vi "SVA 4MV6 PF CCE MGLD PMJD.vi"() -> ()   [LabVIEW 2020]
uses:
  <vilib>/userDefined/High Color/IMAQdx.ctl
  SVA 4MV6 PF CCE MGLD PMJD.ctl
  <vilib>/vision/driver/IMAQdx.llb/IMAQdx Buffer Number Mode.ctl
  <vilib>/vision/driver/NI_Vision_Acquisition_Software.lvlib
panel:
  out "Sin abolladuras":bool
  out "Etiqueta detectada":bool
  out "Orientacion etiqueta correcta":bool
  out "Pass Status":bool
  out "Tapa y etiqueta correctas":bool
  out "Color 2":u32(colorbox)
  out "Color":u32(colorbox)
  out "Color etiqueta":string
  out "Color tapa":string
  out "Nivel de liquido":bool[](array[boolean])
  out "Tapa detectada":bool
  out "Entrada de video":T1(plugin-control)
  out "captura":T1(plugin-control)
  in  "capturar imagen":bool
  in  "stop":bool
  in  "Session In":T2="cam1"
  # "Ceballos Conde Emanuel  Meneses Gutiérrez Luis David  Pineda Méndez Job Daniel\n                            4MV6 Sistemas de vision artificial  Proyecto Final"
  # "Condiciones para Aceptar el producto:\n-Detectar tapa y etiqueta \n-Color de tapa y etiqueta iguales\n-Orientacion de la etiqueta correcta\n-Nivel de liquido dentro del rango maximo\n-Botella sin abolladuras"
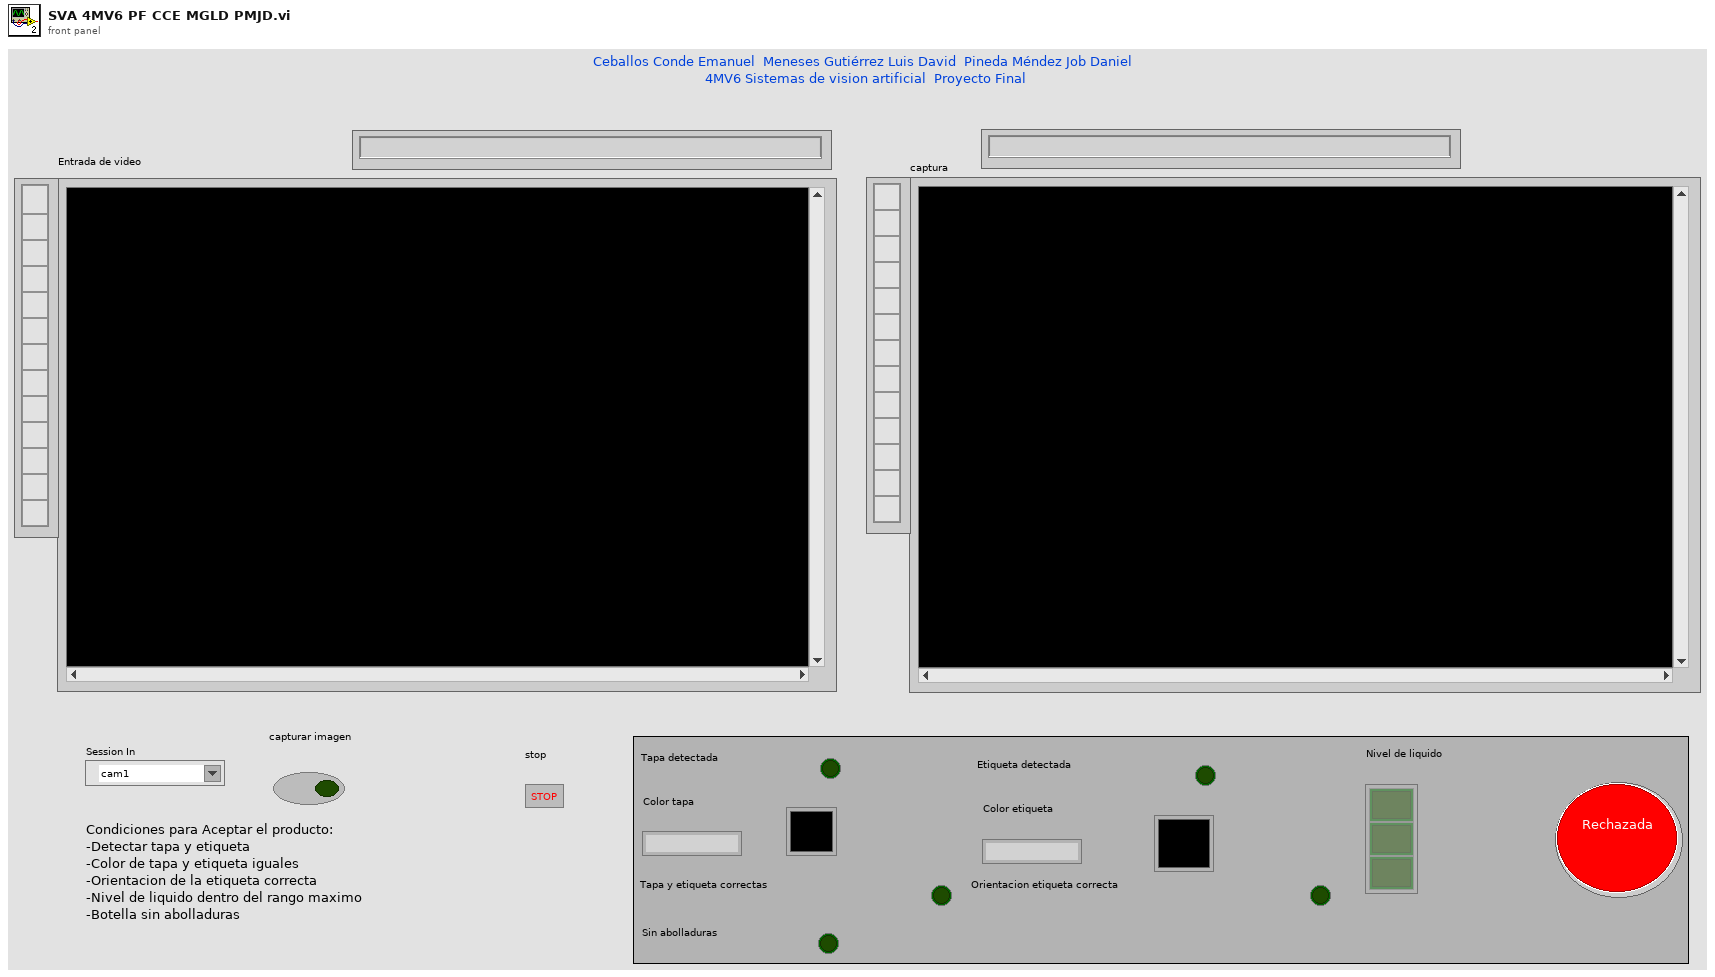
[diagram p1: front panel]
types:
  T1 = typedef "IMAQ Image.ctl" = refnum<image>
  T2 = typedef "IMAQdx.ctl" = refnum<k21>
  T3 = typedef "Image Type" = u32
  T4 = typedef "SVA 4MV6 PF CCE MGLD PMJD.ctl" = enum16{"espera", "captura", "tapa ", "etiqueta", "color", "nivel", "forma", "aceptar"}
  T5 = typedef "NI_Vision_Acquisition_Software.lvlib/IMAQdx Buffer Number Mode.ctl" = enum32{"Next", "Last", "Buffer Number", "Every", "Last New"}
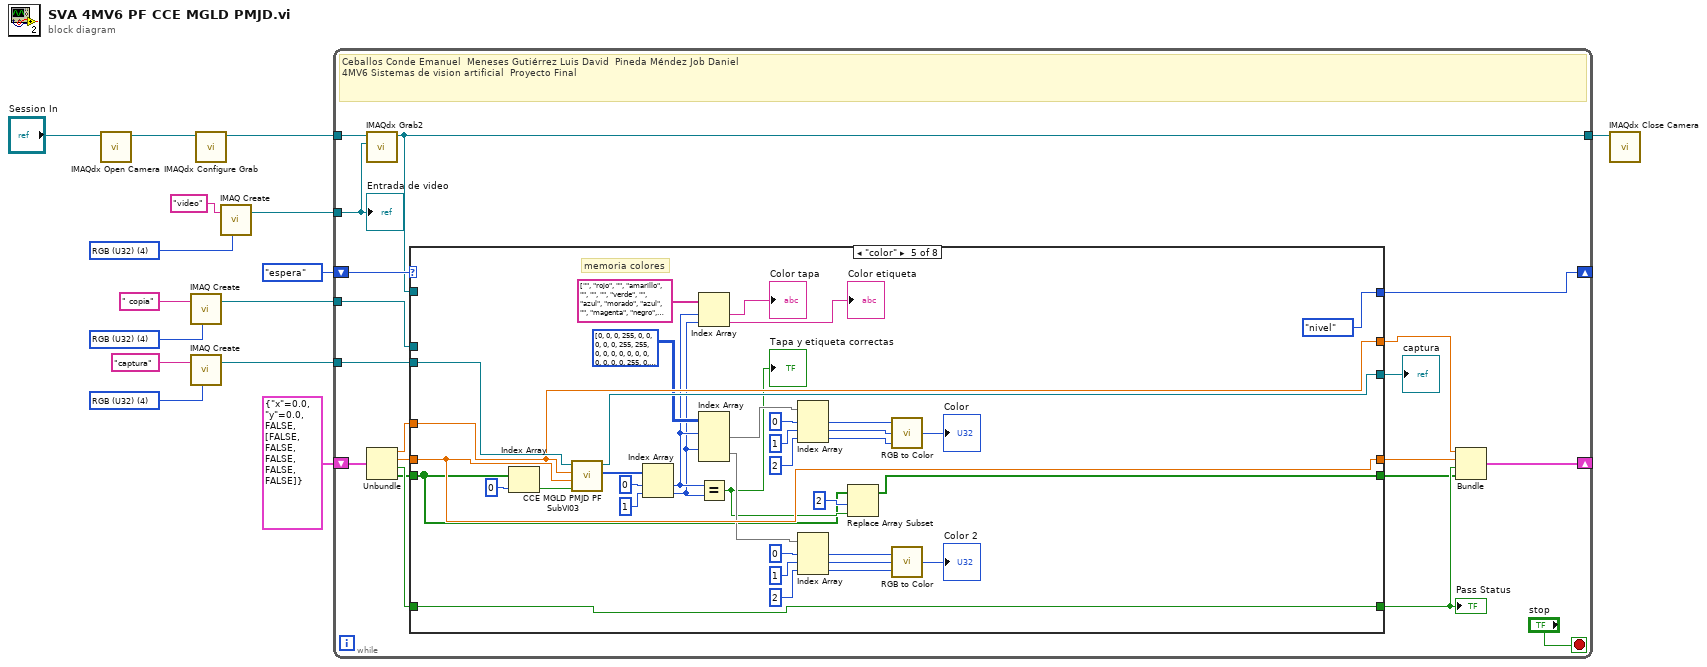
[diagram p0: block diagram]
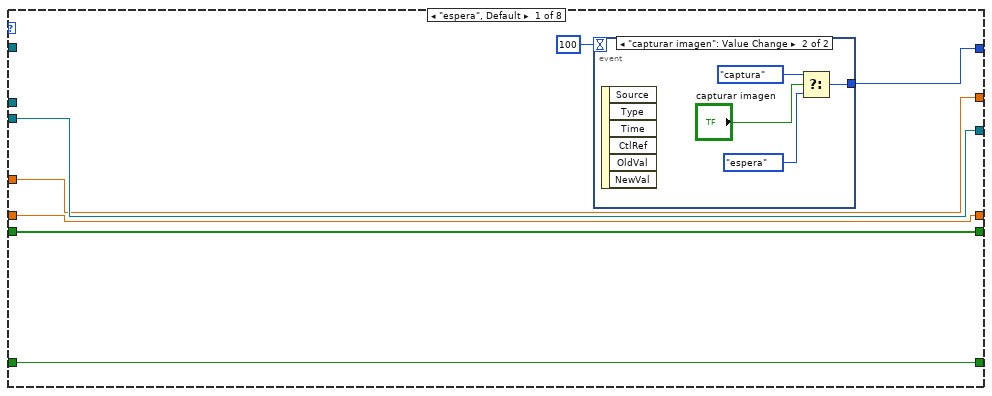
[diagram p2: hidden frame]
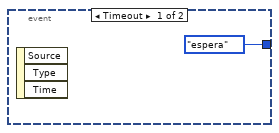
[diagram p3: hidden frame]
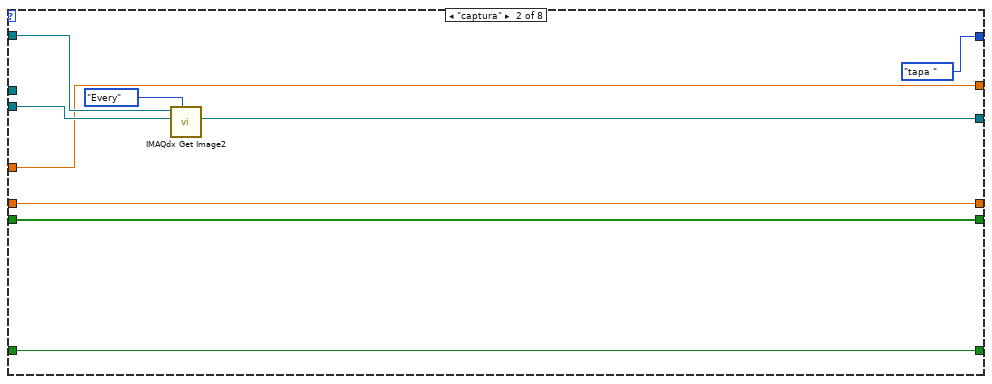
[diagram p4: hidden frame]
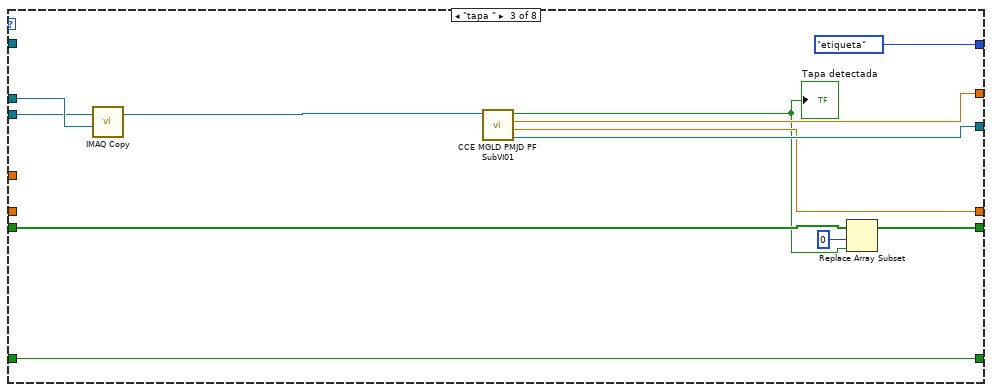
[diagram p5: hidden frame]
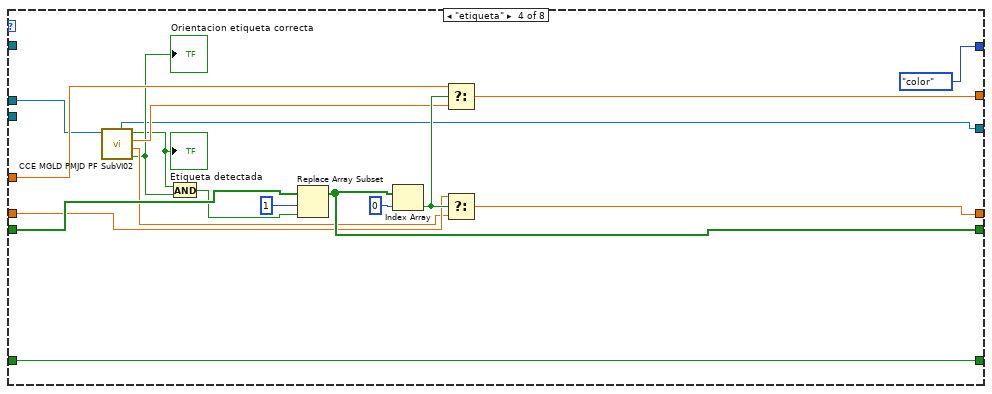
[diagram p6: hidden frame]
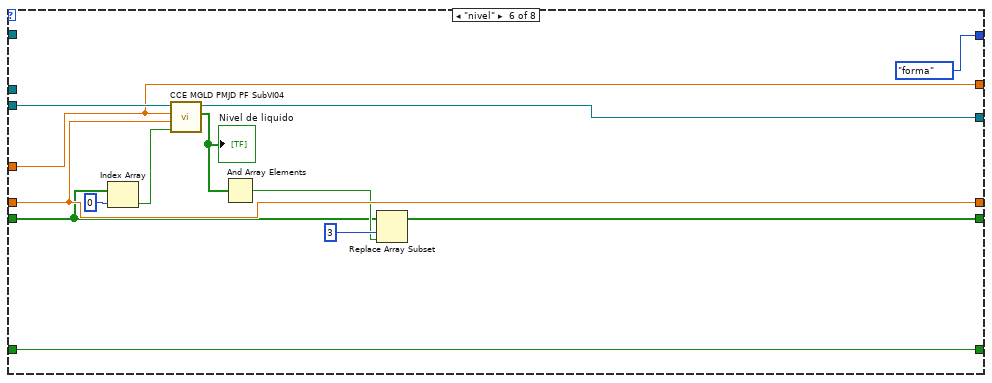
[diagram p7: hidden frame]
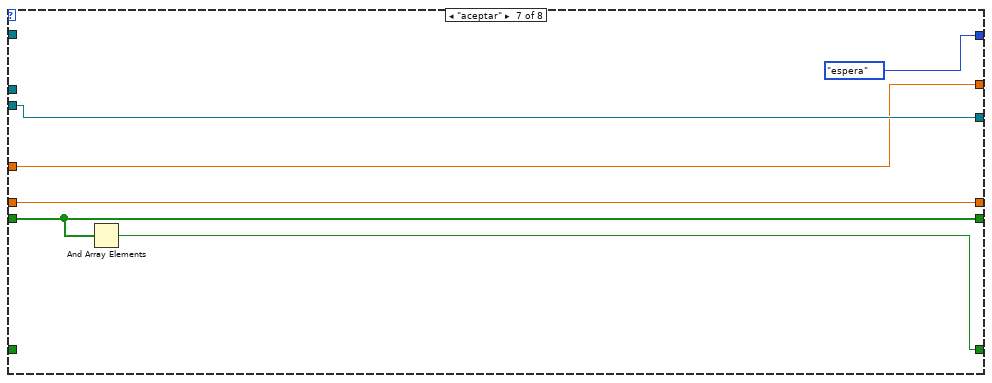
[diagram p8: hidden frame]
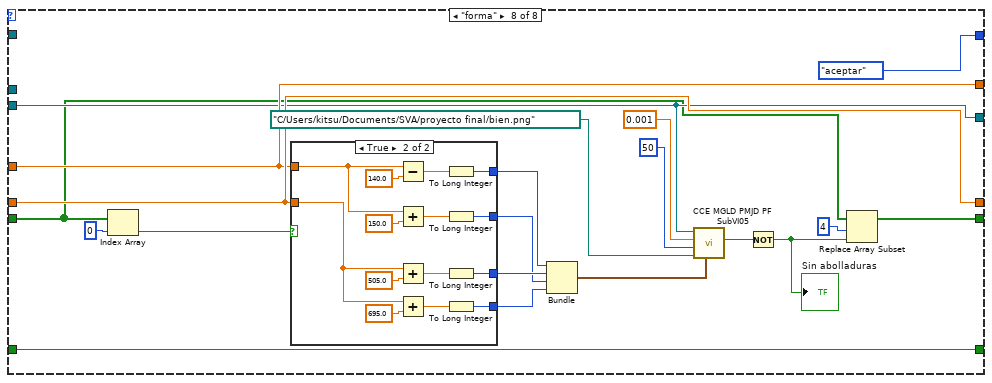
[diagram p9: hidden frame]
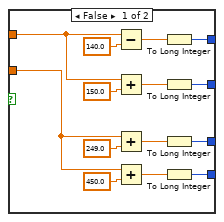
[diagram p10: hidden frame]
diagram:
  w3 = T3 4 items=["Grayscale (U8)", "Grayscale (I16)", "Grayscale (SGL)", "Complex (CSG)", "RGB (U32)", "HSL (U32)", "RGB (U64)", "Grayscale (U16)"] ("Image Type")
  w10 = T3 4 items=["Grayscale (U8)", "Grayscale (I16)", "Grayscale (SGL)", "Complex (CSG)", "RGB (U32)", "HSL (U32)", "RGB (U64)", "Grayscale (U16)"] ("Image Type")
  w12 = T3 4 items=["Grayscale (U8)", "Grayscale (I16)", "Grayscale (SGL)", "Complex (CSG)", "RGB (U32)", "HSL (U32)", "RGB (U64)", "Grayscale (U16)"] ("Image Type")
  n1 = call <vilib>:"IMAQdx Open Camera.vi"("Session In"="Session In") -> ("Session Out"=w14:T2)  [unwired: 9 in, 1 out]
  n2 = call "IMAQ Create"("Image Name"=" copia", "Image Type"=w3) -> ("New Image"=w2:T1)  [unwired: 3 in, 1 out]
  n3 = call "IMAQ Create"("Image Name"="captura", "Image Type"=w12) -> ("New Image"=w5:T1)  [unwired: 3 in, 1 out]
  n4 = call <vilib>:"IMAQdx Configure Grab.vi"("Session In"=w14) -> ("Session Out"=w7:T2)  [unwired: 9 in, 1 out]
  n5 = call "IMAQ Create"("Image Name"="video", "Image Type"=w10) -> ("New Image"=w8:T1)  [unwired: 3 in, 1 out]
  n6 = while {
    shift-right: [w33] -> _
    shift-left: SVA_4MV6_PF_CCE_MGLD_PMJD."espera" -> [w34]
    tunnel: w8 -> [w28]
    tunnel: w7 -> [w32]
    tunnel: [w31] -> w6
    tunnel: w5 -> [w29]
    tunnel: w2 -> [w27]
    shift-right: [w26] -> _
    shift-left: cluster{"x":sgl, "y":sgl, bool, bool[]} {"x"=0.0, "y"=0.0, FALSE, [FALSE, FALSE, FALSE, FALSE, FALSE]} -> [w25]
    stop <- "stop" stop-if-true
    # "Ceballos Conde Emanuel  Meneses Gutiérrez Luis David  Pineda Méndez Job Daniel\n4MV6 Sistemas de vision artificial  Proyecto Final"
    n7 = call <vilib>:"IMAQdx Grab2.vi"("Image In"=w28, "Session In"=w32) -> ("Session Out"=w31:T2)  [unwired: 6 in, 3 out]
    n8 = Unbundle(w25) -> ("x"=w24:sgl, "y"=w23:sgl, w19:bool, w18:bool[])
    n9 = case shown="\"color\"" w34 {
      tunnel: [w40 SVA_4MV6_PF_CCE_MGLD_PMJD."tapa " SVA_4MV6_PF_CCE_MGLD_PMJD."etiqueta" SVA_4MV6_PF_CCE_MGLD_PMJD."color" SVA_4MV6_PF_CCE_MGLD_PMJD."nivel" SVA_4MV6_PF_CCE_MGLD_PMJD."forma" SVA_4MV6_PF_CCE_MGLD_PMJD."espera" SVA_4MV6_PF_CCE_MGLD_PMJD."aceptar"] -> w33
      tunnel: w31 -> [_ w54 _ _ _ _ _ _]
      tunnel: [w39 w53 w66 w70 w121 w132 w140 w150] -> w30
      tunnel: w29 -> [w39 w52 w64 _ w122 w135 w140 w150]
      tunnel: w27 -> [_ _ w65 w71 _ _ _ _]
      tunnel: [w38 w50 w63 w69 w120 w134 w139 w151] -> w22
      tunnel: [w37 w49 w62 w83 w119 w133 w138 w152] -> w21
      tunnel: w24 -> [w38 w50 _ w79 w120 w134 w139 w151]
      tunnel: w23 -> [w37 w49 _ w78 w119 w133 w138 w152]
      tunnel: [w36 w48 w61 w68 w93 w130 w137 w153] -> w20
      tunnel: w19 -> [w36 w48 w61 w68 w93 w130 _ w153]
      tunnel: w18 -> [w35 w47 w60 w84 w88 w124 w136 w143]
      tunnel: [w35 w47 w57 w81 w91 w127 w136 w147] -> w17
      frame "espera", Default {
        n10 = event shown="[1] \"capturar imagen\": Value Change" {
          selector: _ -> [_ _]
          dyn-events: _ -> [_ _]
          timeout: 100 -> [_ _]
          tunnel: [SVA_4MV6_PF_CCE_MGLD_PMJD."espera" w45] -> w40
          event Timeout {
            n11 = event-data() -> ()  [unwired: 1 in, 3 out]
          }
          event "capturar imagen": Value Change {
            n12 = event-data() -> ()  [unwired: 1 in, 6 out]
            n13 = Select(t=SVA_4MV6_PF_CCE_MGLD_PMJD."captura", s="capturar imagen", f=SVA_4MV6_PF_CCE_MGLD_PMJD."espera") -> (s? t:f=w45:T4)
          }
        }
      }
      frame "captura" {
        n14 = call <vilib>:"IMAQdx Get Image2.vi"("Buffer Number Mode (Next)"=IMAQdx_Buffer_Number_Mode."Every", "Image In"=w52, "Session In"=w54) -> ("Image Out"=w53:T1)  [unwired: 5 in, 3 out]
      }
      frame "tapa " {
        n15 = call "IMAQ Copy"("Image Dst"=w65, "Image Src"=w64) -> ("Image Dst Out"=w67:T1)  [unwired: 4 in, 1 out]
        n16 = call "CCE MGLD PMJD PF SubVI01.vi"("captura"=w67) -> ("Image 4"=w66:T1, "y"=w62:sgl, "x"=w63:sgl, "tapa detectada"=w59:bool)  [unwired: 7 in]
        "Tapa detectada" <- w59
        n17 = Replace Array Subset(array=w60, new element=w59, index=0) -> (w57:bool[])
      }
      frame "etiqueta" {
        n18 = call "CCE MGLD PMJD PF SubVI02.vi"("captura"=w71) -> ("orientacion correcta"=w75:bool, "y"=w76:sgl, "x"=w77:sgl, "etiqueta detectada"=w74:bool, "Image 4"=w70:T1)  [unwired: 6 in]
        "Orientacion etiqueta correcta" <- w75
        "Etiqueta detectada" <- w74
        n19 = And(x=w74, y=w75) -> (x .and. y?=w73:bool)
        n20 = Replace Array Subset(array=w84, new element=w73, index=1) -> (w81:bool[])
        n21 = Index Array(array=w81, index=0) -> (element=w82:bool)
        n22 = Select(t=w79, s=w82, f=w77) -> (s? t:f=w69:sgl)
        n23 = Select(t=w78, s=w82, f=w76) -> (s? t:f=w83:sgl)
      }
      frame "color" {
        # "memoria colores"
        n24 = Index Array(array=w88, index=0) -> (element=w87:bool)
        n25 = call "CCE MGLD PMJD PF SubVI03.vi"("tapa?"=w87, "y"=w119, "x"=w120, "Image 2"=w122) -> ("Array"=w94:i32[], "Image"=w121:T1)  [unwired: 6 in]
        n26 = Index Array(array=w94, index #1=0 ("index"), index #2=1 ("index")) -> (element #1=w96:i32, element #2=w95:i32)
        n27 = Index Array(array=string[] ["", "rojo", "", "amarillo", "", "", "", "verde", "", "azul", "morado", "azul", "", "magenta", "negro", "blanco"], index #1=w96, index #2=w95) -> (element #1=→"Color tapa":string, element #2=→"Color etiqueta":string)
        n28 = Index Array(array=u8[][] [[0, 0, 0], [255, 0, 0], [0, 0, 0], [255, 255, 0], [0, 0, 0], [0, 0, 0], [0, 0, 0], [0, 255, 0], [0, 0, 0], [0, 0, 255], [255, 0, 255], [0, 0, 255], [0, 0, 0], [255, 0, 255], [0, 0, 0], [255, 255, 255]], index (row) #1=w96, index (row) #2=w95) -> (element #1=w112:u8[], element #2=w111:u8[])  [unwired: 2 in]
        n29 = Equal?(x=w96, y=w95) -> (x = y?=w90:bool)
        "Tapa y etiqueta correctas" <- w90
        n30 = Index Array(array=w112, index #1=0 ("index"), index #2=1 ("index"), index #3=2 ("index")) -> (element #1=w103:u8, element #2=w102:u8, element #3=w101:u8)
        n31 = Index Array(array=w111, index #1=0 ("index"), index #2=1 ("index"), index #3=2 ("index")) -> (element #1=w99:u8, element #2=w98:u8, element #3=w97:u8)
        n32 = Replace Array Subset(array=w88, new element=w90, index=2) -> (w91:bool[])
        n33 = call <vilib>:"RGB to Color.vi"("B"=w101, "G"=w102, "R"=w103) -> ("Color"=→"Color":u32)
        n34 = call <vilib>:"RGB to Color.vi"("B"=w97, "G"=w98, "R"=w99) -> ("Color"=→"Color 2":u32)
      }
      frame "nivel" {
        n35 = Index Array(array=w124, index=0) -> (element=w125:bool)
        n36 = call "CCE MGLD PMJD PF SubVI04.vi"("tapa?"=w125, "y"=w133, "x"=w134, "Image 2"=w135) -> ("Array"=w131:bool[], "Image"=w132:T1)  [unwired: 6 in]
        "Nivel de liquido" <- w131
        n37 = And Array Elements(Boolean array=w131) -> (logical AND=w128:bool)
        n38 = Replace Array Subset(array=w124, new element=w128, index=3) -> (w127:bool[])
      }
      frame "aceptar" {
        n39 = And Array Elements(Boolean array=w136) -> (logical AND=w137:bool)
      }
      frame "forma" {
        n40 = Index Array(array=w143, index=0) -> (element=w142:bool)
        n41 = case shown="True" w142 {
          tunnel: [w171 w185] -> w161
          tunnel: [w166 w180] -> w160
          tunnel: [w165 w179] -> w159
          tunnel: [w164 w178] -> w158
          tunnel: w152 -> [w163 w177]
          tunnel: w151 -> [w162 w176]
          frame False {
            n42 = Subtract(x=w162, y=sgl 140.0) -> (x-y=w175:sgl)
            n43 = Add(x=w162, y=sgl 150.0) -> (x+y=w172:sgl)
            n44 = Add(x=w163, y=sgl 249.0) -> (x+y=w174:sgl)
            n45 = Add(x=w163, y=sgl 450.0) -> (x+y=w173:sgl)
            n46 = To Long Integer(number=w175) -> (32bit integer=w171:i32)
            n47 = To Long Integer(number=w172) -> (32bit integer=w165:i32)
            n48 = To Long Integer(number=w174) -> (32bit integer=w166:i32)
            n49 = To Long Integer(number=w173) -> (32bit integer=w164:i32)
          }
          frame True {
            n50 = Subtract(x=w176, y=sgl 140.0) -> (x-y=w189:sgl)
            n51 = Add(x=w176, y=sgl 150.0) -> (x+y=w186:sgl)
            n52 = Add(x=w177, y=sgl 505.0) -> (x+y=w188:sgl)
            n53 = Add(x=w177, y=sgl 695.0) -> (x+y=w187:sgl)
            n54 = To Long Integer(number=w189) -> (32bit integer=w185:i32)
            n55 = To Long Integer(number=w186) -> (32bit integer=w179:i32)
            n56 = To Long Integer(number=w188) -> (32bit integer=w180:i32)
            n57 = To Long Integer(number=w187) -> (32bit integer=w178:i32)
          }
        }
        n58 = Bundle(w161, w160, w159, w158) -> (w157:cluster{i32, i32, i32, i32})  [unwired: 1 in]
        n59 = call "CCE MGLD PMJD PF SubVI05.vi"("Coordenadas"=w157, "DireccionMemoria"=path "C:/Users/kitsu/Documents/SVA/proyecto final/bien.png", "UMBRAL"=u8 50, "Tolerancia"=0.001, "Image"=w150) -> ("Abolladuas?"=w146:bool)  [unwired: 5 in, 1 out]
        n60 = Not(x=w146) -> (.not. x?=w145:bool)
        "Sin abolladuras" <- w145
        n61 = Replace Array Subset(array=w143, new element=w145, index=4) -> (w147:bool[])
      }
    }
    "captura" <- w30
    "Pass Status" <- w20
    n62 = Bundle("x"=w22, "y"=w21, w20, w17) -> (w26:cluster{"x":sgl, "y":sgl, bool, bool[]})  [unwired: 1 in]
    "Entrada de video" <- w28
  }
  n63 = call <vilib>:"IMAQdx Close Camera.vi"("Session In"=w6) -> ()  [unwired: 10 in, 1 out]
